vi "DSF.Engine.Memory.Cache.Transfer Group.Get Transfer Cache.vi"(10 "Transfer ID":i32, 11 "Transfer Group Cache in":refnum<class "DSF.Engine.Memory.Cache.Transfer Group.lvclass">) -> (2 "Transfer Cache":refnum<class "DSF.Engine.Memory.Cache.Transfer.lvclass">, 3 "Transfer Group Cache out":refnum<class "DSF.Engine.Memory.Cache.Transfer Group.lvclass">)   [LabVIEW 2017, in "DSF.Engine.lvlib" / "DSF.Engine.Memory.Cache.Transfer Group.lvclass"]
uses:
  DSF.Engine.Memory.Cache.Transfer Group.lvclass
  DSF.Engine.Memory.Cache.Transfer.lvclass
  DSF.Engine.Memory.Cache.Transfer Group.lvclass/DSF.Engine.Memory.Cache.Transfer Group.ctl
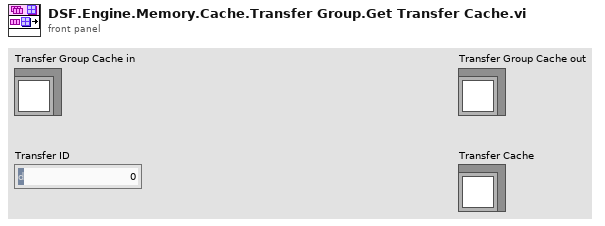
[diagram p1: front panel]
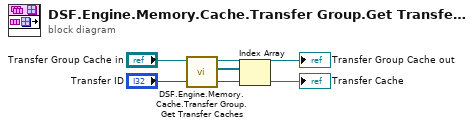
[diagram p0: block diagram]
diagram:
  n1 = call "DSF.Engine.Memory.Cache.Transfer Group.Get Transfer Caches.vi"("Transfer Group Cache in"="Transfer Group Cache in") -> ("Transfer Caches"=w4:refnum<class "DSF.Engine.Memory.Cache.Transfer.lvclass">[], "Transfer Group Cache out"=→"Transfer Group Cache out":refnum<class "DSF.Engine.Memory.Cache.Transfer Group.lvclass">)  [unwired: 9 in]
  n2 = Index Array(array=w4, index="Transfer ID") -> (element=→"Transfer Cache":refnum<class "DSF.Engine.Memory.Cache.Transfer.lvclass">)
